vi "PS Control Write.vi"(0 "Magnet System":enum16{"Resistive", "Hybrid"}(ring), 1 "Ramp":bool=TRUE, 7 "Setpoint":dbl format="%.2f", 11 "error in (no error)":errorcluster) -> (4 "Time(ms)":u32, 15 "error out":errorcluster)   [LabVIEW 2019]
panel:
  out "State":T1(ring)=enum."Set-STOP"
  # "(To Zero Goes\nTo 100 A)"
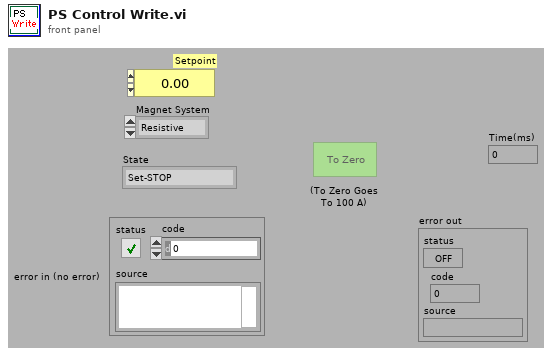
[diagram p1: front panel]
types:
  T1 = enum16{"--Quit--", "Set-STOP", "Set-Pause", "Set-FRTZ", "Set-Ramp", "Set-Setpoint"}
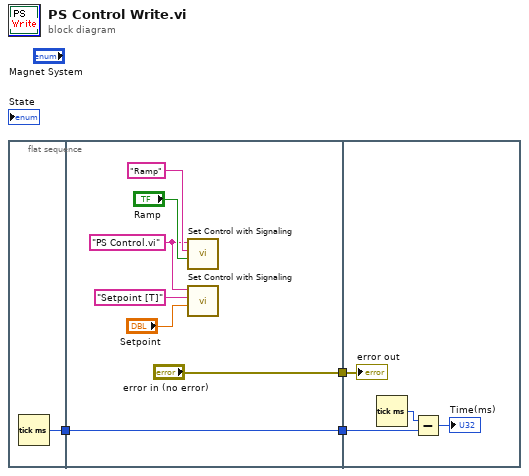
[diagram p0: block diagram]
diagram:
  n1 = flat-sequence {
    tunnel: [w4] -> w2
    tunnel: [w6] -> w3
    tunnel: w2 -> [w6]
    tunnel: ["error in (no error)"] -> w1
    tunnel: w3 -> [w13]
    tunnel: w1 -> [w12]
    frame #0 {
      n2 = Tick Count (ms)() -> (millisecond timer value=w4:u32)
    }
    frame #1 {
      w9 = "PS Control.vi"
      n3 = call "Set Control with Signaling.vi"("Value"="Ramp", "Control Name"="Ramp", "VI Name"=w9) -> ()  [unwired: 8 in, 1 out]
      n4 = call "Set Control with Signaling.vi"("Value"="Setpoint", "Control Name"="Setpoint [T]", "VI Name"=w9) -> ()  [unwired: 8 in, 1 out]
    }
    frame #2 {
      n5 = Tick Count (ms)() -> (millisecond timer value=w14:u32)
      n6 = Subtract(x=w14, y=w13) -> (x-y=→"Time(ms)":u32)
      "error out" <- w12
    }
  }
